vi "UBX_Paser.vi"() -> ()   [LabVIEW 2015]
uses:
  <vilib>/Instr/_visa.llb/VISA Configure Serial Port (Instr).vi
panel:
  out "GPS_KHP":dbl
  in  "Baud Rate":u32=115200
  in  "정지":bool
  out "X(lat)":dbl format="%-#_10g M"
  out "Y(long)":dbl format="%-#_10g M"
  out "F9P_Data_GPGGA_Raw":string
  in  "ms 배수":u32=20
  out "*(타입 *) &x":T1
  out "Heading_M":dbl
  out "Heading_T":dbl
  out "F9P GPS Data":T2
  in  "COM":refnum<visa-resource-name>="COM12"
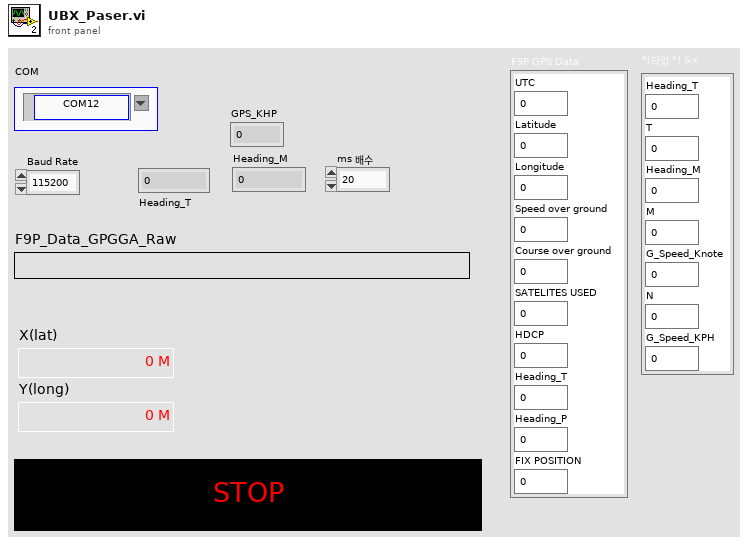
[diagram p1: front panel]
types:
  T1 = cluster{"Heading_T":dbl, "T":i8, "Heading_M":dbl, "M":i8, "G_Speed_Knote":dbl, "N":i8, "G_Speed_KPH":dbl}
  T2 = cluster{"UTC":dbl, "Latitude":dbl, "Longitude":dbl, "Speed over ground":dbl, "Course over ground":dbl, "SATELITES USED":i32, "HDCP":dbl, "Heading_T":dbl, "Heading_P":dbl, "FIX POSITION":i32}
  T3 = cluster{"X(lat)":dbl, "Y(long)":dbl, "Heading_T":dbl, "Heading_M":dbl, "GPS_SPD(kph)":dbl}
  T4 = cluster{"UTC":dbl, "Latitude":dbl, "N/S":i8, "Longitude":dbl, "N/S":i8, "FIX POSITION":i32, "SATELITES USED":i32, "HDCP":dbl}
  T5 = cluster{"UTC":dbl, "N/S":i8, "Latitude":dbl, "N/S 2":i8, "Longitude":dbl, "N/S 3":i8, "Speed over ground":dbl, "Course over ground":dbl}
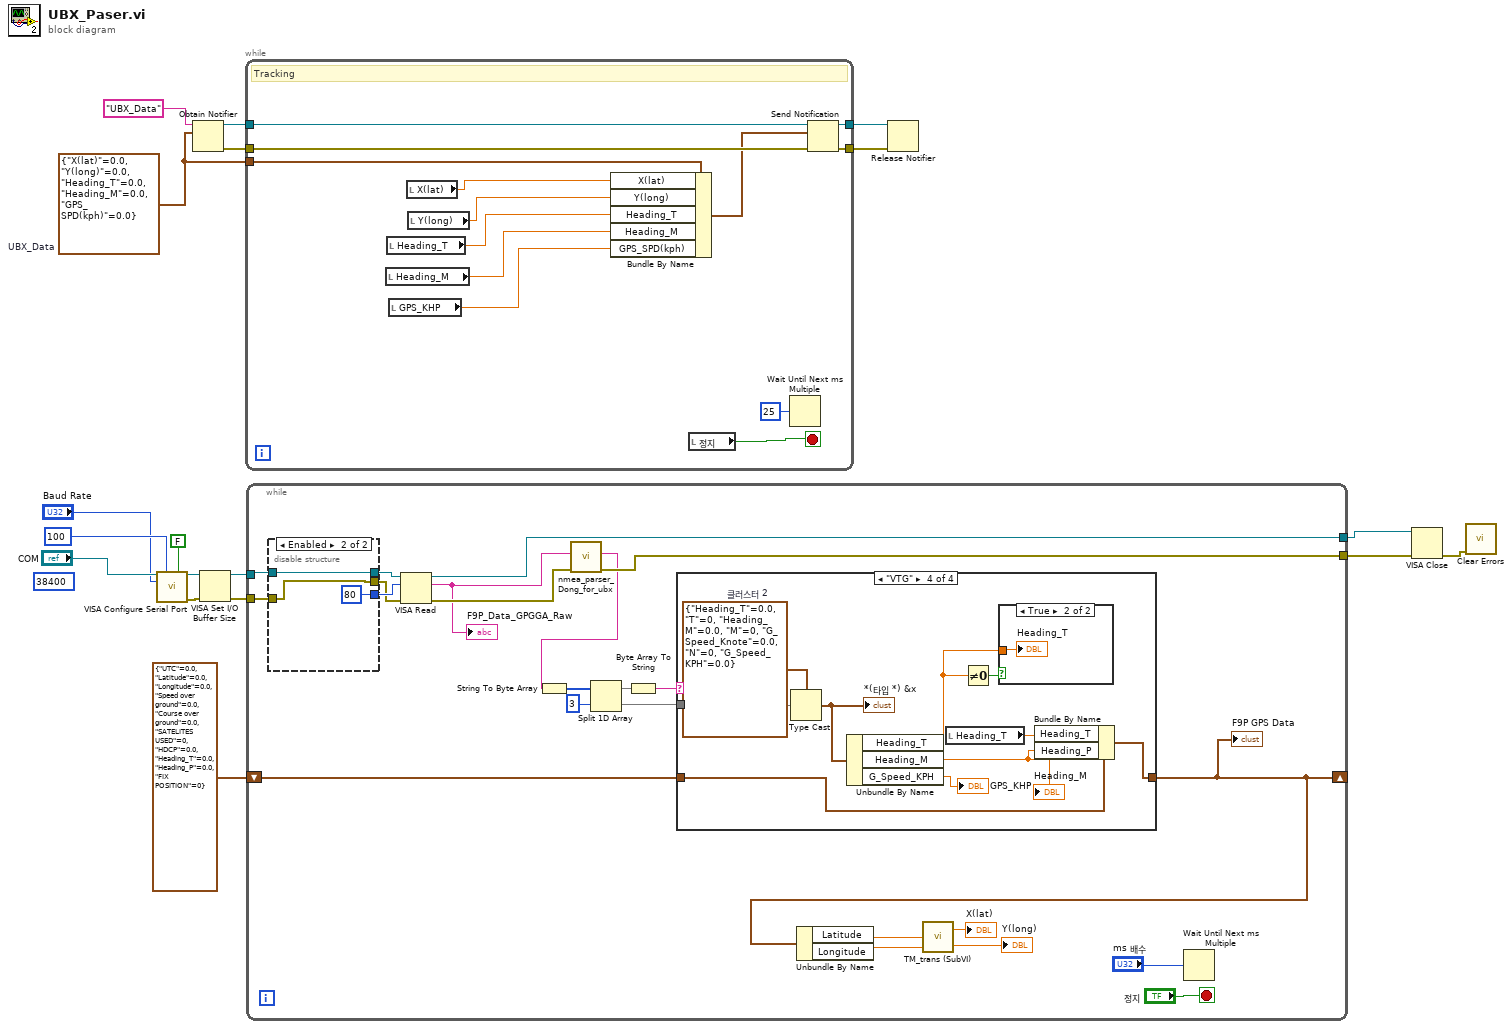
[diagram p0: block diagram]
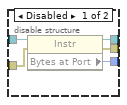
[diagram p2: hidden frame]
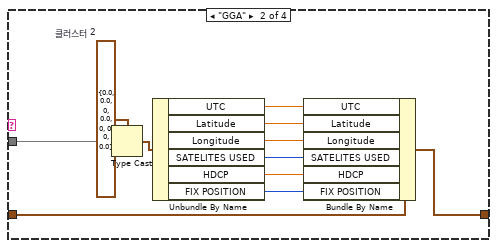
[diagram p4: hidden frame]
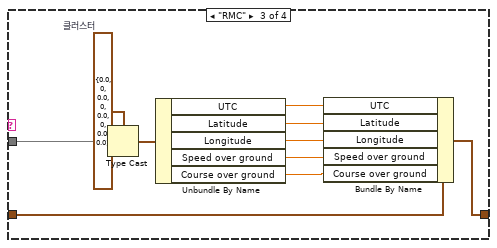
[diagram p5: hidden frame]
diagram:
  w1 = T3 {"X(lat)"=0.0, "Y(long)"=0.0, "Heading_T"=0.0, "Heading_M"=0.0, "GPS_SPD(kph)"=0.0}  # UBX_Data
  (unwired) u32 38400 ("baud rate")
  n1 = call-poly "VISA Configure Serial Port"("VISA resource name"="COM", "timeout (10sec)"=u32 100, "Enable Termination\nChar (T)"=FALSE ("Enable Termination\nChar (T)"), "baud rate (9600)"="Baud Rate") -> ("VISA resource name out"=w15:refnum<visa-resource-name>, "error out"=w14:errorcluster)  [unwired: 10 in]
  n2 = Obtain Notifier(name (unnamed)="UBX_Data" ("이름(이름없음)"), notification data type=w1) -> (notifier out=w5:refnum<notifier>, error out=w4:errorcluster)  [unwired: 2 in, 1 out]
  n3 = VISA Set I/O Buffer Size(VISA resource name=w15, error in (no error)=w14) -> (VISA resource name out=w9:refnum<visa-resource-name>, error out=w8:errorcluster)  [unwired: 2 in]
  n4 = while {
    tunnel: w5 -> [w30]
    tunnel: w4 -> [w28]
    tunnel: [w27] -> w3
    tunnel: [w29] -> w2
    tunnel: w1 -> [w26]
    stop <- w24 stop-if-true
    # "Tracking"
    n5 = local read "Heading_M"() -> (w20:dbl)
    n6 = local read "Heading_T"() -> (w21:dbl)
    n7 = local read "GPS_KHP"() -> (w19:dbl)
    n8 = local read "X(lat)"() -> (w22:dbl)
    n9 = local read "Y(long)"() -> (w23:dbl)
    n10 = Bundle By Name(cluster=w26, "X(lat)"=w22, "Y(long)"=w23, "Heading_T"=w21, "Heading_M"=w20, "GPS_SPD(kph)"=w19) -> (w25:T3)
    n11 = local read "정지"() -> (w24:bool)
    n12 = Wait Until Next ms Multiple(millisecond multiple=u32 25) -> ()  [unwired: 1 out]
    n13 = Send Notification(notification=w25, notifier=w30, error in (no error)=w28) -> (notifier out=w29:refnum<notifier>, error out=w27:errorcluster)
  }
  n14 = while {
    shift-right: [w44] -> _
    shift-left: T2 {"UTC"=0.0, "Latitude"=0.0, "Longitude"=0.0, "Speed over ground"=0.0, "Course over ground"=0.0, "SATELITES USED"=0, "HDCP"=0.0, "Heading_T"=0.0, "Heading_P"=0.0, "FIX POSITION"=0} ("Garmin GPS Data") -> [w53]
    tunnel: w9 -> [w36]
    tunnel: w8 -> [w34]
    tunnel: [w45] -> w13
    tunnel: [w52] -> w12
    stop <- "정지" stop-if-true
    n15 = disable-structure shown="Enabled" {
      disable-tunnel: [w59 u32 80 ("Bytes at Port")] -> w37
      disable-tunnel: w36 -> [w58 w61]
      disable-tunnel: [w57 w61] -> w35
      disable-tunnel: w34 -> [w56 w60]
      disable-tunnel: [w55 w60] -> w32
      frame Disabled {
        n16 = property class="Instr"(reference=w58, error in=w56) -> (reference out=w57:refnum<visa-resource-name>, error out=w55:errorcluster, "Bytes at Port"=w59:u32)
      }
      frame Enabled {
      }
    }
    n17 = VISA Read(VISA resource name=w35, byte count=w37, error in (no error)=w32) -> (VISA resource name out=w45:refnum<visa-resource-name>, read buffer=w46:string, error out=w51:errorcluster)  [unwired: 1 out]
    "F9P_Data_GPGGA_Raw" <- w46
    n18 = call "nmea_parser_Dong_for_ubx.vi"("error in"=w51, "INPUT"=w46) -> ("error out"=w52:errorcluster, "output"=w38:string)  [unwired: 8 in]
    n19 = String To Byte Array(string=w38) -> (unsigned byte array=w42:u8[])
    n20 = Split 1D Array(array=w42, index=3) -> (first subarray=w41:u8[], second subarray=w40:u8[])
    n21 = Byte Array To String(unsigned byte array=w41) -> (string=w39:string)
    n22 = case shown="\"VTG\"" w39 {
      tunnel: w40 -> [_ w74 w82 w94]
      tunnel: w53 -> [w63 w70 w81 w89]
      tunnel: [w63 w69 w80 w90] -> w44
      frame Default {
      }
      frame "GGA" {
        w72 = T4 {"UTC"=0.0, "Latitude"=0.0, "N/S"=0, "Longitude"=0.0, "N/S"=0, "FIX POSITION"=0, "SATELITES USED"=0, "HDCP"=0.0}  # 클러스터 2
        n23 = Type Cast(type=w72, x=w74) -> (*(type *) &x=w73:T4)
        n24 = Unbundle By Name(w73) -> ("UTC"=w71:dbl, "Latitude"=w68:dbl, "Longitude"=w67:dbl, "SATELITES USED"=w66:i32, "HDCP"=w65:dbl, "FIX POSITION"=w64:i32)
        n25 = Bundle By Name(cluster=w70, "UTC"=w71, "Latitude"=w68, "Longitude"=w67, "SATELITES USED"=w66, "HDCP"=w65, "FIX POSITION"=w64) -> (w69:T2)
      }
      frame "RMC" {
        w84 = T5 {"UTC"=0.0, "N/S"=0, "Latitude"=0.0, "N/S 2"=0, "Longitude"=0.0, "N/S 3"=0, "Speed over ground"=0.0, "Course over ground"=0.0}  # 클러스터
        n26 = Type Cast(type=w84, x=w82) -> (*(type *) &x=w83:T5)
        n27 = Unbundle By Name(w83) -> ("UTC"=w79:dbl, "Latitude"=w78:dbl, "Longitude"=w77:dbl, "Speed over ground"=w76:dbl, "Course over ground"=w75:dbl)
        n28 = Bundle By Name(cluster=w81, "UTC"=w79, "Latitude"=w78, "Longitude"=w77, "Speed over ground"=w76, "Course over ground"=w75) -> (w80:T2)
      }
      frame "VTG" {
        w93 = T1 {"Heading_T"=0.0, "T"=0, "Heading_M"=0.0, "M"=0, "G_Speed_Knote"=0.0, "N"=0, "G_Speed_KPH"=0.0}  # 클러스터 2
        n29 = Type Cast(type=w93, x=w94) -> (*(type *) &x=w92:T1)
        "*(타입 *) &x" <- w92
        n30 = Unbundle By Name(w92) -> ("Heading_T"=w88:dbl, "Heading_M"=w91:dbl, "G_Speed_KPH"=→"GPS_KHP":dbl)
        "Heading_M" <- w91
        n31 = local read "Heading_T"() -> (w86:dbl)
        n32 = Not Equal To 0?(x=w88) -> (x != 0?=w87:bool)
        n33 = case shown="True" w87 {
          tunnel: w88 -> [_ w95]
          frame False {
          }
          frame True {
            "Heading_T" <- w95
          }
        }
        n34 = Bundle By Name(cluster=w89, "Heading_T"=w86, "Heading_P"=w91) -> (w90:T2)
      }
    }
    "F9P GPS Data" <- w44
    n35 = Unbundle By Name(w44) -> ("Latitude"=w50:dbl, "Longitude"=w49:dbl)
    n36 = call "TM_trans (SubVI).vi"("long"=w49, "lat"=w50) -> ("Y(long)"=→"Y(long)":dbl, "X(lat)"=→"X(lat)":dbl)  [unwired: 1 in]
    n37 = Wait Until Next ms Multiple(millisecond multiple="ms 배수") -> ()  [unwired: 1 out]
  }
  n38 = Release Notifier(notifier=w2, error in (no error)=w3) -> ()  [unwired: 1 in, 3 out]
  n39 = VISA Close(VISA resource name=w13, error in (no error)=w12) -> (error out=w7:errorcluster)
  n40 = call <vilib>:"Clear Errors.vi"("error in (no error)"=w7) -> ()  [unwired: 5 in, 2 out]
